vi "Setup Start Collect.vi"(8 "error in (no error)":errorcluster, 9 "Lasers ON?":bool, 10 "Wait Notifier":refnum<notifier>, 11 "Move Length":i32) -> (0 "error out":errorcluster, 2 "Success":bool)   [LabVIEW 2015, in "Collect Data Mgr.lvlib"]
uses:
  Collect Data Mgr.lvlib
  Start Collect (Reply Payload)--cluster.ctl
  Tool Interface/Tool Interface.lvlib
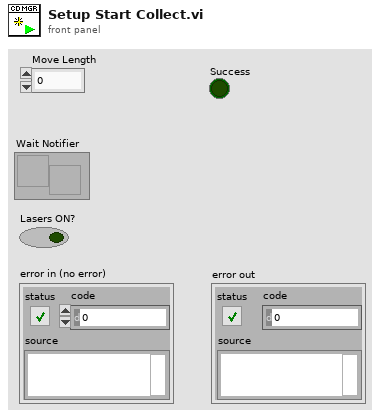
[diagram p1: front panel]
types:
  T1 = typedef "Collect Data Mgr.lvlib/Start Collect (Reply Payload)--cluster.ctl" = cluster{"Success":bool, "CD_Status":u8}
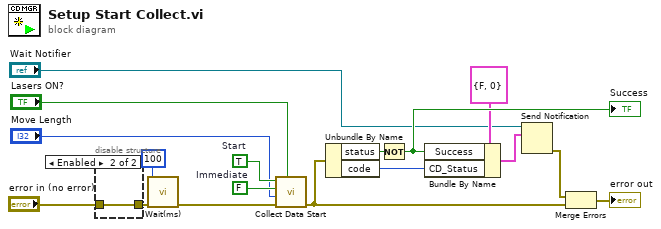
[diagram p0: block diagram]
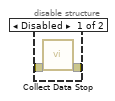
[diagram p2: hidden frame]
diagram:
  w9 = FALSE  # Immediate
  w10 = TRUE  # Start
  n1 = disable-structure shown="Enabled" {
    disable-tunnel: [w19 w20] -> w12
    disable-tunnel: "error in (no error)" -> [w18 w20]
    frame Disabled {
      n2 = call "Collect Data Stop.vi"("error in (no error)"=w18) -> ("error out"=w19:errorcluster)  [unwired: 10 in]
    }
    frame Enabled {
    }
  }
  n3 = call "Wait(ms).vi"("error in (no error)"=w12, "milliseconds"=u32 100) -> ("error out"=w4:errorcluster)  [unwired: 9 in]
  n4 = call "Collect Data Start.vi"("Lasers ON?"="Lasers ON?", "error in (no error)"=w4, "Length"="Move Length", "Immediate"=w9, "Start"=w10) -> ("error out"=w8:errorcluster)  [unwired: 6 in]
  n5 = Unbundle By Name(w8) -> ("status"=w16:bool, "code"=w13:i32)
  n6 = Not(x=w16) -> (.not. x?=w17:bool)
  "Success" <- w17
  n7 = Bundle By Name(cluster=T1 {"Success"=FALSE, "CD_Status"=0} ("Start Collect (Reply Payload)"), "Success"=w17, "CD_Status"=w13) -> (w14:T1)
  n8 = Send Notification(notification=w14, notifier="Wait Notifier") -> (error out=w7:errorcluster)  [unwired: 1 in, 1 out]
  n9 = Merge Errors(w7, w8) -> (→"error out":errorcluster)
